vi "通知器 多对一通信.vi"() -> ()   [LabVIEW 2011]
uses:
  <userlib>/_OpenG.lib/numeric/numeric.llb/Random Number Within Range - DBL__ogtk.vi
panel:
  out "notifier name":string
  out "notifications":string[](array[string])
  in  "stop 2":bool
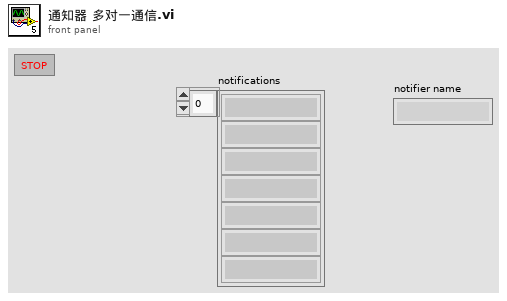
[diagram p1: front panel]
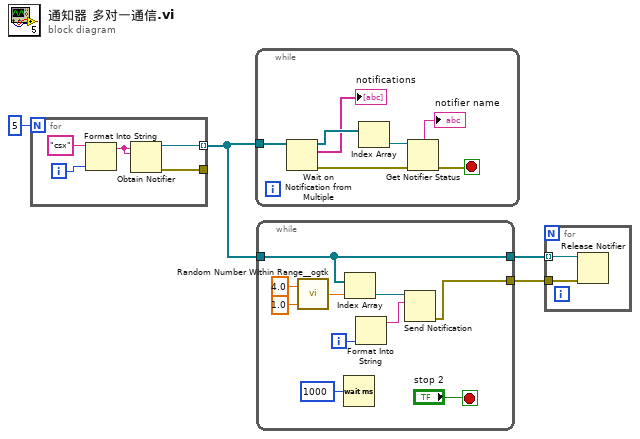
[diagram p0: block diagram]
diagram:
  n1 = for {
    N: 5 -> [_]
    tunnel: [w9] -> w4 mode=indexing
    tunnel: [w8] -> _
    i -> [w5]
    n2 = Format Into String(initial string="csx" ("name (unnamed)"), w5) -> (resulting string=w6:string)  [unwired: 2 in, 1 out]
    n3 = Obtain Notifier(name (unnamed)=w6, notification data type=w6) -> (notifier out=w9:refnum<notifier>, error out=w8:errorcluster)  [unwired: 2 in, 1 out]
  }
  n4 = while {
    tunnel: w4 -> [w16]
    stop <- w10 stop-if-true
    n5 = Wait on Notification from Multiple(0:w16) -> (8:w15:refnum<notifier>[], 9:→"notifications":string[], 11:w11:errorcluster)  [unwired: 3 in, 1 out]
    n6 = Index Array(array=w15) -> (element=w13:refnum<notifier>)  [unwired: 1 in]
    n7 = Get Notifier Status(notifier=w13, error in (no error)=w11) -> (notifier name=→"notifier name":string, error out=w10:errorcluster)  [unwired: 3 out]
  }
  n8 = while {
    tunnel: w4 -> [w18]
    tunnel: [w18] -> w3
    tunnel: [w17] -> w2
    i -> [w21]
    stop <- "stop 2" stop-if-true
    n9 = call-poly <userlib>:"Random Number Within Range__ogtk.vi"("High"=4.0, "Low"=1.0) -> ("Random Number"=w25:dbl)  [unwired: 3 in]
    n10 = Wait (ms)(milliseconds to wait=u32 1000) -> ()  [unwired: 1 out]
    n11 = Index Array(array=w18, index=w25) -> (element=w22:refnum<notifier>)
    n12 = Format Into String(w21) -> (resulting string=w20:string)  [unwired: 3 in, 1 out]
    n13 = Send Notification(notification=w20, notifier=w22) -> (error out=w17:errorcluster)  [unwired: 1 in, 1 out]
  }
  n14 = for {
    tunnel: w3 -> [w28] mode=indexing
    tunnel: w2 -> [w27]
    n15 = Release Notifier(notifier=w28, error in (no error)=w27) -> ()  [unwired: 1 in, 3 out]
  }
